vi "energia_moc.vi"(11 "signal in":waveform(dbl)) -> (2 "Numeric":dbl, 3 "Numeric 2":dbl)   [LabVIEW 2025]
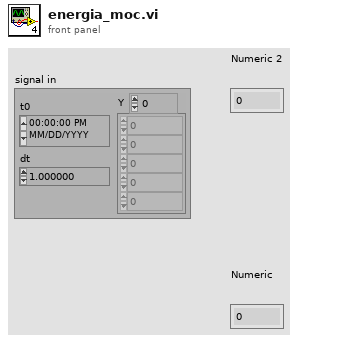
[diagram p1: front panel]
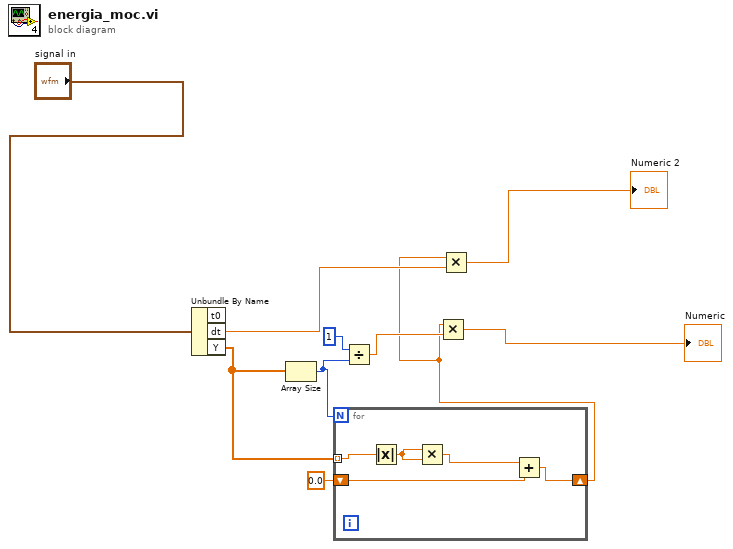
[diagram p0: block diagram]
diagram:
  n1 = Unbundle By Name("signal in") -> ("dt"=w3:dbl, "Y"=w6:dbl[])  [unwired: 1 out]
  n2 = Array Size(array=w6) -> (size(s)=w7:i32)
  n3 = for {
    N: w7 -> [_]
    shift-right: [w14] -> w2
    shift-left: 0.0 -> [w15]
    tunnel: w6 -> [w13] mode=indexing
    n4 = Absolute Value(x=w13) -> (abs(x)=w12:dbl)
    n5 = Multiply(x=w12, y=w12) -> (x*y=w11:dbl)
    n6 = Add(x=w11, y=w15) -> (x+y=w14:dbl)
  }
  n7 = Divide(x=1, y=w7) -> (x/y=w8:dbl)
  n8 = Multiply(x=w2, y=w8) -> (x*y=→"Numeric":dbl)
  n9 = Multiply(x=w2, y=w3) -> (x*y=→"Numeric 2":dbl)
